vi "Broadcast Exposure Time.vi"(8 "error in (no error)":errorcluster, 10 "Reply Payload":T1) -> (0 "error out":errorcluster)   [LabVIEW 2020, in "Camera.lvlib"]
doc: "Set the exposure time in seconds. The exposure time returned is the exposure time actually set by in the device.\n_____\nCreated using Delacor QMH Event Scripter 5.0.0.112."
uses:
  Camera.lvlib
  Set Accumulations (Reply Payload)--cluster.ctl
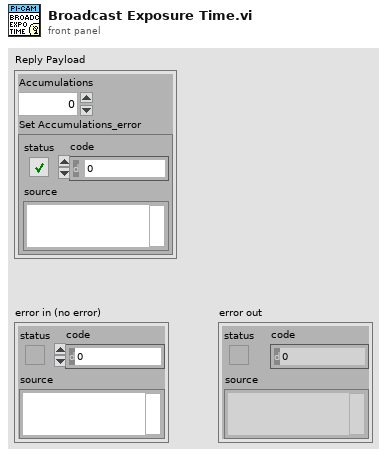
[diagram p1: front panel]
types:
  T1 = typedef "Camera.lvlib/Set Accumulations (Reply Payload)--cluster.ctl" = cluster{"Accumulations":i64, "Set Accumulations_error":errorcluster}
  T2 = typedef "Camera.lvlib/Broadcast Events--cluster.ctl" = cluster{"Module Did Init":refnum<user-event>, "Status Updated":refnum<user-event>, "Error Reported":refnum<user-event>, "Module Did Stop":refnum<user-event>, "Update Module Execution Status":refnum<user-event>, "Broadcast Image":refnum<user-event>, "Broadcast Exposure Time":refnum<user-event>, "Broadcast Binning":refnum<user-event>, "Broadcast GatingMode":refnum<user-event>, "Broadcast RepetitiveGate":refnum<user-event>, "Broadcast IntensifierStatus":refnum<user-event>, "Broadcast IntensifierGain":refnum<user-event>, "Broadcast EMIccdGainControlMode":refnum<user-event>, "Broadcast EMIccdGain":refnum<user-event>, "Broadcast FloatingPoint Parameter":refnum<user-event>, "Broadcast Integer Parameter":refnum<user-event>, "Broadcast LargeInteger Parameter":refnum<user-event>, "Broadcast Pulse Parameter":refnum<user-event>, "Broadcast SensorTemperatureStatus":refnum<user-event>}
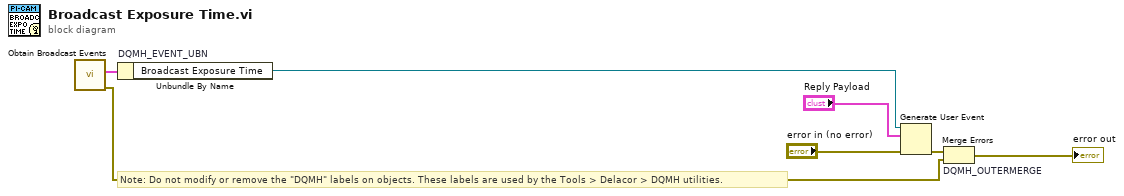
[diagram p0: block diagram]
diagram:
  # "Note: Do not modify or remove the \"DQMH\" labels on objects. These labels are used by the Tools > Delacor > DQMH utilities."
  n1 = call "Obtain Broadcast Events.vi"() -> ("error out"=w2:errorcluster, "Camera Broadcast Events"=w1:T2)  [unwired: 10 in]
  n2 = Unbundle By Name "DQMH_EVENT_UBN"(w1) -> ("Broadcast Exposure Time"=w4:refnum<user-event>)
  n3 = Generate User Event(user event=w4, event data cluster="Reply Payload", error in="error in (no error)") -> (error out=w3:errorcluster)  [unwired: 1 in, 1 out]
  n4 = Merge Errors "DQMH_OUTERMERGE"(w3, w2) -> (→"error out":errorcluster)
